vi "HWIO Send API Command.vi"(0 "Action":string, 1 "Timeout ms (5000)":i32=5000, 5 "Double":dbl[](array[numeric]), 7 "Integer":i32[](array[numeric]), 9 "Boolean":bool[](array[boolean]), 11 "String":string[](array[string]), 12 "error in (no error)":errorcluster) -> (3 "Timed Out?":bool, 4 "Action out":string, 6 "Double out":dbl[](array[numeric]), 8 "Integer out":i32[](array[numeric]), 10 "Boolean out":bool[](array[boolean]), 13 "HWError":errorcluster, 14 "error out":errorcluster, 15 "String out":string[](array[string]))   [LabVIEW 2011]
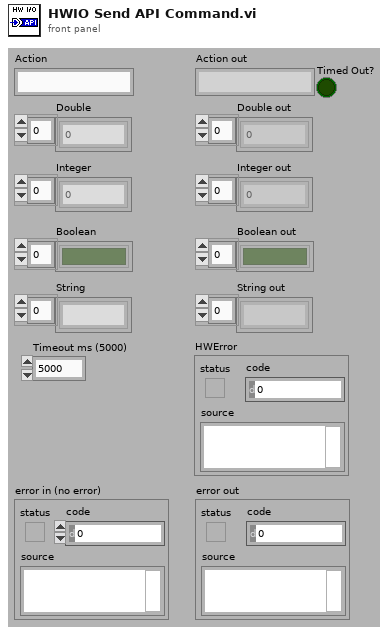
[diagram p1: front panel]
types:
  T1 = typedef "PIM.API.Command.Unique.ctl" = cluster{"#attributes":cluster{"Action":string}, "Double":dbl[], "Integer":i32[], "Boolean":bool[], "String":string[]}
  T2 = typedef "PIM.API.Response.Unique.ctl" = cluster{"#attributes":cluster{"Action":string, "Units":string}, "Double":dbl[], "Integer":i32[], "Boolean":bool[], "String":string[], "Sample":T3[], "Status":cluster{"#attributes":cluster{"Error":bool, "Code":i32}, "Message":string}[]}
  T3 = typedef "PIM.API.Response.Samples.ctl" = cluster{"TX1":cluster{"#attributes":cluster{"Frequency":dbl, "Power_dBm":dbl, "Power_Watts":dbl, "CheckTx":bool, "Unleveled":bool, "Squelched":bool, "Temperature":dbl, "ToneOn":bool}}, "TX2":cluster{"#attributes":cluster{"Frequency":dbl, "Power_dBm":dbl, "Power_Watts":dbl, "CheckTx":bool, "Unleveled":bool, "Squelched":bool, "Temperature":dbl, "ToneOn":bool}}, "IM":cluster{"#attributes":cluster{"Frequency":dbl, "Power_dBm":dbl, "PeakPower_dBm":dbl, "Power_dBc":dbl, "PeakPower_dBc":dbl, "IM_Order":u8, "IM Overload":bool}}[], "#attributes":cluster{"Count":u32, "Total":u32, "Finished?":bool, "Sweep Leg":T4, "F1":dbl, "F2":dbl, "FStep":dbl}}
  T4 = typedef "iQA Sweep Behavior.ctl" = enum16{"F2Down", "F1Up", "RxMultiIM"}
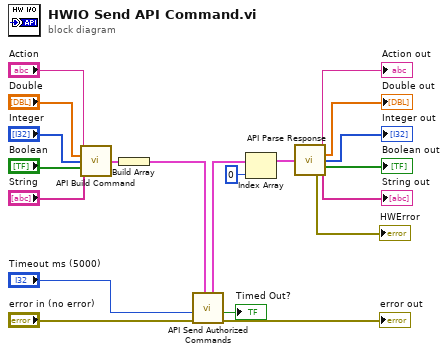
[diagram p0: block diagram]
diagram:
  n1 = call "API Build Command.vi"("Action"="Action", "Double"="Double", "Integer"="Integer", "Boolean"="Boolean", "String"="String") -> ("PIM.API.Command.Unique"=w18:T1)  [unwired: 10 in]
  n2 = Build Array(w18) -> (w5:T1[])
  n3 = call "API Send Authorized Commands.vi"("Commands"=w5, "error in (no error)"="error in (no error)", "Timeout ms (5000)"="Timeout ms (5000)") -> ("error out"=→"error out":errorcluster, "Timed Out?"=→"Timed Out?":bool, "Responses"=w4:T2[])  [unwired: 6 in]
  n4 = Index Array(array=w4, index=0) -> (element=w20:T2)
  n5 = call "API Parse Response.vi"("PIM.API.Response.Unique"=w20) -> ("Action"=→"Action out":string, "Double"=→"Double out":dbl[], "Integer"=→"Integer out":i32[], "Boolean"=→"Boolean out":bool[], "error out"=→"HWError":errorcluster, "String"=→"String out":string[])  [unwired: 8 in, 1 out]
